vi "ConfigurationPage.vi"(9 "Parameter defaults":string, 10 "Parameters":T1, 11 "Stop":T2) -> ()   [LabVIEW 2020, in "DefaultExtensions.lvlib" / "CDefaultRuleFileParser.lvclass"]
uses:
  CDefaultRuleFileParser.lvclass
  obj/Addons/ExtensionInterfaces.lvlibp/IConfigurationPage/Event_StopRef.ctl
  obj/Addons/ExtensionInterfaces.lvlibp/IConfigurationPage/Event_Stop.ctl
  obj/Addons/ExtensionInterfaces.lvlibp/IConfigurationPage/Event_ParametersRef.ctl
  obj/Addons/ExtensionInterfaces.lvlibp/IConfigurationPage/Event_Parameters.ctl
  Private/Paramters.ctl
  obj/Addons/ExtensionInterfaces.lvlibp/IConfigurationPage/IConfigurationPage.lvclass
panel:
  in  "Rules file path":path
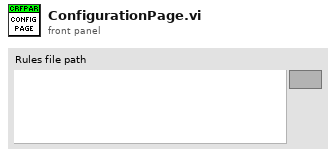
[diagram p1: front panel]
types:
  T1 = typedef "ExtensionInterfaces.lvlibp/IConfigurationPage.lvclass/Event_ParametersRef.ctl" = refnum<user-event>
  T2 = typedef "ExtensionInterfaces.lvlibp/IConfigurationPage.lvclass/Event_StopRef.ctl" = refnum<user-event>
  T3 = typedef "DefaultExtensions.lvlib/CDefaultRuleFileParser.lvclass/Paramters.ctl" = cluster{"Path":string}
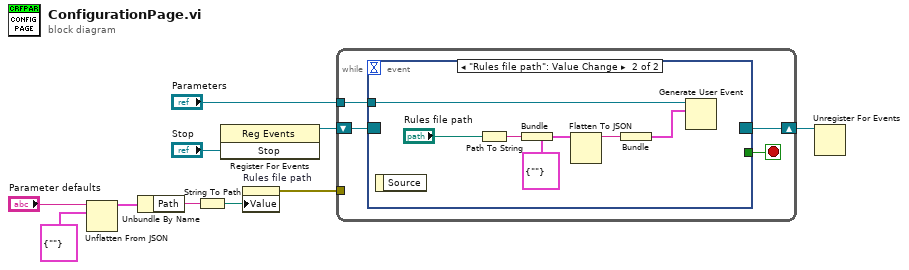
[diagram p0: block diagram]
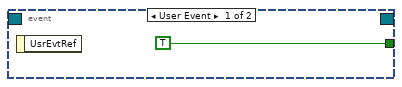
[diagram p2: hidden frame]
diagram:
  n1 = Unflatten From JSON(JSON string="Parameter defaults", type and defaults=T3 {"Path"=""} ("Parameters")) -> (value=w4:T3)  [unwired: 5 in, 1 out]
  n2 = Unbundle By Name(w4) -> ("Path"=w3:string)
  n3 = String To Path(string=w3) -> (path=w2:path)
  n4 = register-events("Stop") -> (reference out=w10:refnum<event-registration>)  [unwired: 2 in, 1 out]
  n5 = property on="Rules file path" class="Path"("Value"=w2) -> (error out=w1:errorcluster)  [unwired: 2 in, 1 out]
  n6 = while {
    shift-right: [w13] -> w9
    shift-left: w10 -> [w14]
    tunnel: "Parameters" -> [w11]
    tunnel: w1 -> [_]
    stop <- w12 stop-if-true
    n7 = event shown="[1] \"Rules file path\": Value Change" {
      selector: w14 -> [_ _]
      dyn-events: [_ _] -> w13
      timeout: _ -> [_ _]
      tunnel: [TRUE _] -> w12
      tunnel: w11 -> [_ w18]
      event User Event {
        n8 = event-data() -> ()  [unwired: 1 in, 1 out]
      }
      event "Rules file path": Value Change {
        n9 = event-data() -> ()  [unwired: 1 in, 1 out]
        n10 = Path To String(path="Rules file path") -> (string=w21:string)
        n11 = Bundle(cluster=T3 {"Path"=""} ("Parameters"), "Path"=w21) -> (w22:T3)
        n12 = Flatten To JSON(anything=w22) -> (JSON string=w20:string)  [unwired: 2 in, 1 out]
        n13 = Bundle("JSON string"=w20) -> (w19:cluster{"JSON string":string})  [unwired: 1 in]
        n14 = Generate User Event(user event=w18, event data cluster=w19) -> ()  [unwired: 2 in, 2 out]
      }
    }
  }
  n15 = Unregister For Events(event registration refnum=w9) -> ()  [unwired: 1 in, 1 out]
